vi "repPrepareKickoffAllyPlayVSS.vi"(8 "error in (no error)":errorcluster, 9 "Game in 2":refnum<class "Game.lvclass">, 10 "RobotPlacement":T1(array[cluster]), 11 "PrepareKickoffAllyPlayVSS in":refnum<class "PrepareKickoffAllyPlayVSS.lvclass">) -> (0 "error out":errorcluster, 2 "RobotPlacement 2":T1(array[cluster]), 3 "PrepareKickoffAllyPlayVSS out":refnum<class "PrepareKickoffAllyPlayVSS.lvclass">)   [LabVIEW 2023, in "PrepareKickoffAllyPlayVSS.lvclass"]
uses:
  PrepareKickoffAllyPlayVSS.lvclass
  Game_class/Game.lvclass
  Game_class/Game.lvclass/Game.ctl
  Game_class/Read FieldRef.vi
  Field_class/Field.lvclass
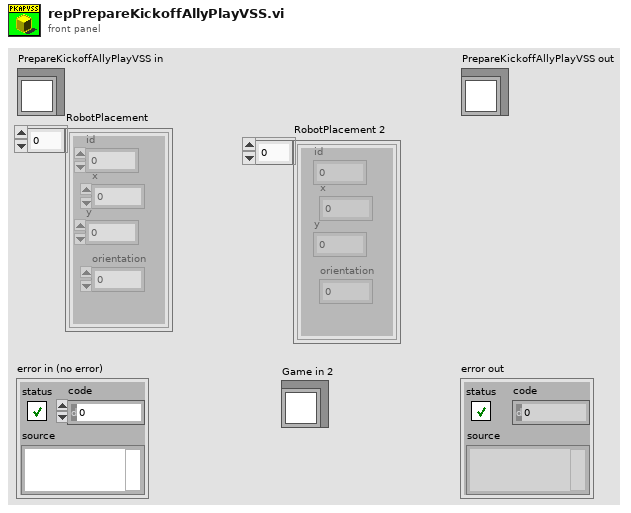
[diagram p1: front panel]
types:
  T1 = cluster{"id":i32, "x":dbl, "y":dbl, "orientation":dbl}[]
  T2 = cluster{"id":i32, "x":dbl, "y":dbl, "orientation":dbl}
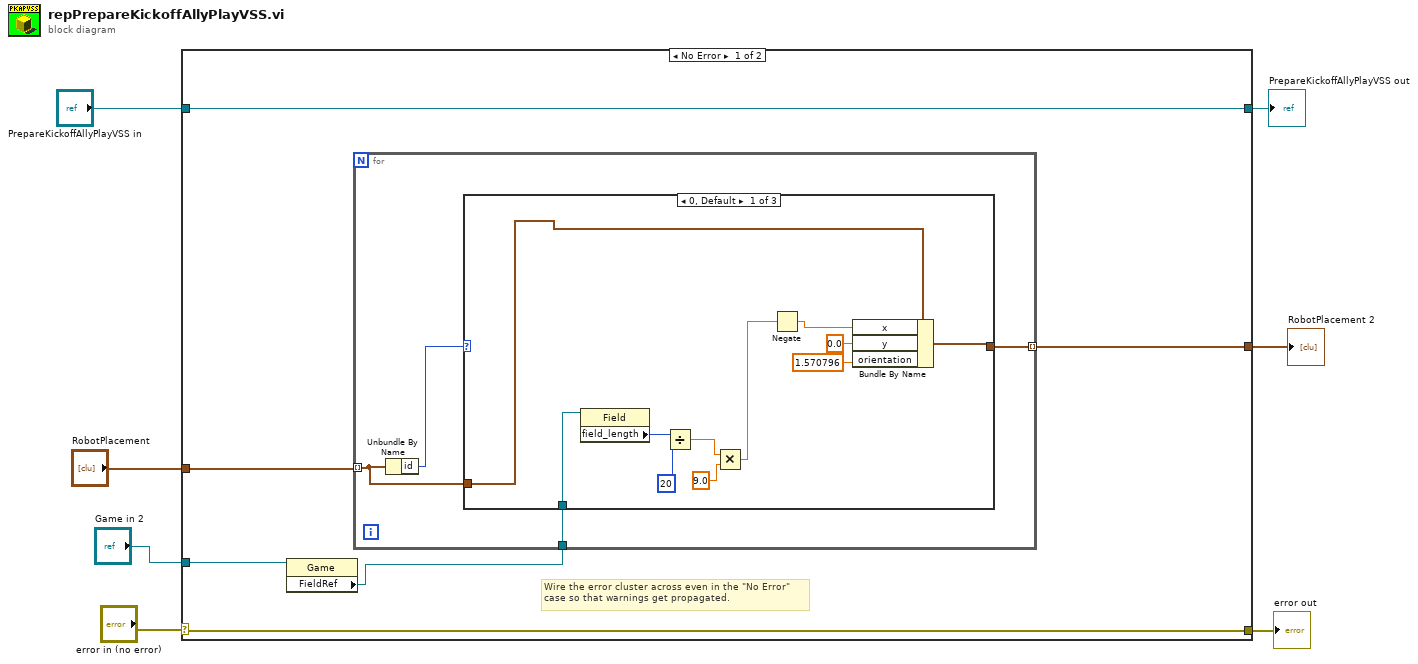
[diagram p0: block diagram]
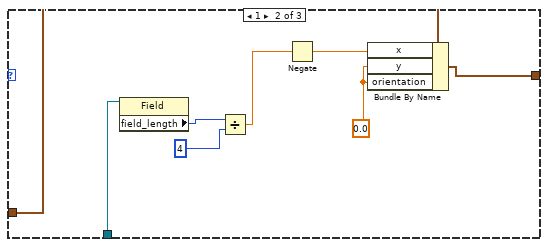
[diagram p2: hidden frame]
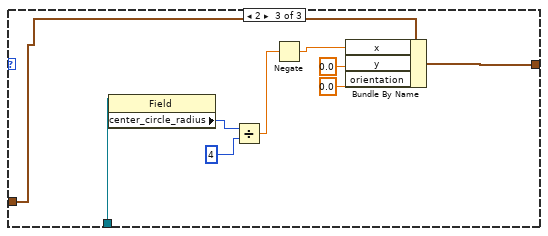
[diagram p3: hidden frame]
diagram:
  n1 = case shown="No Error" "error in (no error)" {
    selector: "error in (no error)" -> [w12 w47]
    tunnel: [w12 w47] -> w6
    tunnel: [w13 w46] -> w4
    tunnel: "PrepareKickoffAllyPlayVSS in" -> [w13 w46]
    tunnel: "RobotPlacement" -> [w11 _]
    tunnel: "Game in 2" -> [w10 _]
    tunnel: [w8 _] -> w1
    frame No Error {
      # "Wire the error cluster across even in the \"No Error\"\ncase so that warnings get propagated."
      n2 = property class="Game"(reference=w10) -> ("FieldRef"=w9:refnum<class "Field.lvclass">)  [unwired: 1 in, 2 out]
      n3 = for {
        tunnel: w11 -> [w16] mode=indexing
        tunnel: [w15] -> w8 mode=indexing
        tunnel: w9 -> [w14]
        n4 = Unbundle By Name(w16) -> ("id"=w17:i32)
        n5 = case shown="0, Default" w17 {
          tunnel: w16 -> [w28 w36 w45]
          tunnel: [w27 w35 w44] -> w15
          tunnel: w14 -> [w26 w33 w41]
          frame 0, Default {
            n6 = property class="Field"(reference=w26) -> ("field_length"=w25:i32)  [unwired: 1 in, 2 out]
            n7 = Divide(x=w25, y=20) -> (x/y=w20:dbl)
            n8 = Multiply(x=w20, y=9.0) -> (x*y=w19:dbl)
            n9 = Negate(x=w19) -> (-x=w21:dbl)
            n10 = Bundle By Name(cluster=w28, "x"=w21, "y"=0.0, "orientation"=1.570796) -> (w27:T2)
          }
          frame 1 {
            w34 = 0.0 ("x")
            n11 = property class="Field"(reference=w33) -> ("field_length"=w31:i32)  [unwired: 1 in, 2 out]
            n12 = Divide(x=w31, y=4) -> (x/y=w30:dbl)
            n13 = Negate(x=w30) -> (-x=w29:dbl)
            n14 = Bundle By Name(cluster=w36, "x"=w29, "y"=w34, "orientation"=w34) -> (w35:T2)
          }
          frame 2 {
            n15 = property class="Field"(reference=w41) -> ("center_circle_radius"=w39:i32)  [unwired: 1 in, 2 out]
            n16 = Divide(x=w39, y=4) -> (x/y=w38:dbl)
            n17 = Negate(x=w38) -> (-x=w37:dbl)
            n18 = Bundle By Name(cluster=w45, "x"=w37, "y"=0.0, "orientation"=0.0) -> (w44:T2)
          }
        }
      }
    }
    frame Error {
    }
  }
  "error out" <- w6
  "PrepareKickoffAllyPlayVSS out" <- w4
  "RobotPlacement 2" <- w1
